vi "Sensoren_buendeln.vi"(0 "rechts seite":dbl, 1 "Links seite":dbl, 2 "Links schräg":dbl, 3 "rechts Schräg":dbl, 4 "rechts geradeaus":dbl, 5 "Links Geradeaus":dbl) -> (14 "SensorArray":dbl[](array[numeric]))   [LabVIEW 2016]
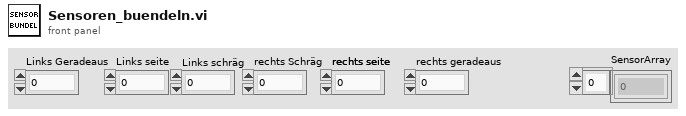
[diagram p1: front panel]
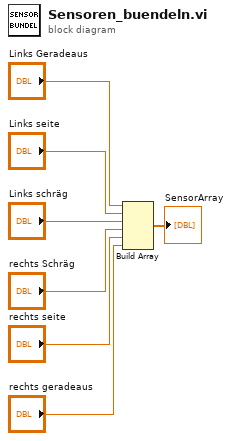
[diagram p0: block diagram]
diagram:
  n1 = Build Array("Links Geradeaus", "Links seite", "Links schräg", "rechts Schräg", "rechts seite", "rechts geradeaus") -> (→"SensorArray":dbl[])
